vi "Main.vi"(7 "sweep rate, /min":dbl=0.2, 8 "sweep to:":dbl=-0.5, 9 "sweep":T3(radio)=enum."time_sweep") -> ()   [LabVIEW 2017] (continued)
                n2113 = property on="data_caption" class="Str"() -> ("Value"=w2662:string)  [unwired: 2 in, 2 out]
                n2114 = case shown="False" w2663 {
                  tunnel: w2662 -> [w2665 w2671]
                  tunnel: [w2665 w2670] -> w2661
                  tunnel: w2660 -> [w2664 w2668]
                  tunnel: [w2664 w2666] -> w2659
                  frame False {
                    # "not measure SR830 2 in phase signal (SR830_2_ip)"
                  }
                  frame True {
                    w2667 = "SR830_2_ip"
                    # "measure SR830 2 in phase signal (SR830_2_ip)"
                    n2115 = local read "SR830 2 addr"() -> (w2672:u8)
                    n2116 = Number To Decimal String(number=w2672) -> (decimal integer string=w2673:string)  [unwired: 1 in]
                    n2117 = GPIB Clear(3:w2673) -> ()  [unwired: 1 in, 2 out]
                    n2118 = Build Array (concatenate)(w2668, w2667) -> (w2666:string[])
                    n2119 = Concatenate Strings(w2671, w2667, "\t") -> (w2670:string)
                  }
                }
                n2120 = property on="Figure_axis" class="Arr (strict)"("Value"=w2659) -> ()  [unwired: 2 in, 2 out]
                n2121 = property on="data_caption" class="Str"("Value"=w2661) -> ()  [unwired: 2 in, 2 out]
              }
              frame #3 {
                # "SR830 2 out of phase (SR830_2_oop)"
                n2122 = local read "SR830 2 oop"() -> (w2678:bool)
                n2123 = property on="Figure_axis" class="Arr (strict)"() -> ("Value"=w2675:string[])  [unwired: 2 in, 2 out]
                n2124 = property on="data_caption" class="Str"() -> ("Value"=w2677:string)  [unwired: 2 in, 2 out]
                n2125 = case shown="False" w2678 {
                  tunnel: w2677 -> [w2680 w2686]
                  tunnel: [w2680 w2685] -> w2676
                  tunnel: w2675 -> [w2679 w2683]
                  tunnel: [w2679 w2681] -> w2674
                  frame False {
                    # "not measure SR830 2 out of phase signal (SR830_2_oop)"
                  }
                  frame True {
                    w2682 = "SR830_2_oop"
                    # "measure SR830 2 out of phase signal (SR830_2_oop)"
                    n2126 = local read "SR830 2 addr"() -> (w2687:u8)
                    n2127 = Number To Decimal String(number=w2687) -> (decimal integer string=w2688:string)  [unwired: 1 in]
                    n2128 = GPIB Clear(3:w2688) -> ()  [unwired: 1 in, 2 out]
                    n2129 = Build Array (concatenate)(w2683, w2682) -> (w2681:string[])
                    n2130 = Concatenate Strings(w2686, w2682, "\t") -> (w2685:string)
                  }
                }
                n2131 = property on="Figure_axis" class="Arr (strict)"("Value"=w2674) -> ()  [unwired: 2 in, 2 out]
                n2132 = property on="data_caption" class="Str"("Value"=w2676) -> ()  [unwired: 2 in, 2 out]
              }
              frame #4 {
                # "SR830 3 in phase (SR830_3_ip)"
                n2133 = local read "SR830 3 ip"() -> (w2693:bool)
                n2134 = property on="Figure_axis" class="Arr (strict)"() -> ("Value"=w2690:string[])  [unwired: 2 in, 2 out]
                n2135 = property on="data_caption" class="Str"() -> ("Value"=w2692:string)  [unwired: 2 in, 2 out]
                n2136 = case shown="False" w2693 {
                  tunnel: w2692 -> [w2695 w2701]
                  tunnel: [w2695 w2700] -> w2691
                  tunnel: w2690 -> [w2694 w2698]
                  tunnel: [w2694 w2696] -> w2689
                  frame False {
                    # "not measure SR830 3 in phase signal (SR830_3_ip)"
                  }
                  frame True {
                    w2697 = "SR830_3_ip"
                    # "measure SR830 3 in phase signal (SR830_3_ip)"
                    n2137 = local read "SR830 3 addr"() -> (w2702:u8)
                    n2138 = Number To Decimal String(number=w2702) -> (decimal integer string=w2703:string)  [unwired: 1 in]
                    n2139 = GPIB Clear(3:w2703) -> ()  [unwired: 1 in, 2 out]
                    n2140 = Build Array (concatenate)(w2698, w2697) -> (w2696:string[])
                    n2141 = Concatenate Strings(w2701, w2697, "\t") -> (w2700:string)
                  }
                }
                n2142 = property on="Figure_axis" class="Arr (strict)"("Value"=w2689) -> ()  [unwired: 2 in, 2 out]
                n2143 = property on="data_caption" class="Str"("Value"=w2691) -> ()  [unwired: 2 in, 2 out]
              }
              frame #5 {
                # "SR830 3 out of phase (SR830_3_oop)"
                n2144 = local read "SR830 3 oop"() -> (w2708:bool)
                n2145 = property on="Figure_axis" class="Arr (strict)"() -> ("Value"=w2705:string[])  [unwired: 2 in, 2 out]
                n2146 = property on="data_caption" class="Str"() -> ("Value"=w2707:string)  [unwired: 2 in, 2 out]
                n2147 = case shown="False" w2708 {
                  tunnel: w2707 -> [w2710 w2716]
                  tunnel: [w2710 w2715] -> w2706
                  tunnel: w2705 -> [w2709 w2713]
                  tunnel: [w2709 w2711] -> w2704
                  frame False {
                    # "not measure SR830 3 out of phase signal (SR830_3_oop)"
                  }
                  frame True {
                    w2712 = "SR830_3_oop"
                    # "measure SR830 3 out phase signal (SR830_3_oop)"
                    n2148 = local read "SR830 3 addr"() -> (w2717:u8)
                    n2149 = Number To Decimal String(number=w2717) -> (decimal integer string=w2718:string)  [unwired: 1 in]
                    n2150 = GPIB Clear(3:w2718) -> ()  [unwired: 1 in, 2 out]
                    n2151 = Build Array (concatenate)(w2713, w2712) -> (w2711:string[])
                    n2152 = Concatenate Strings(w2716, w2712, "\t") -> (w2715:string)
                  }
                }
                n2153 = property on="Figure_axis" class="Arr (strict)"("Value"=w2704) -> ()  [unwired: 2 in, 2 out]
                n2154 = property on="data_caption" class="Str"("Value"=w2706) -> ()  [unwired: 2 in, 2 out]
              }
              frame #6 {
                # "SR830 4 in phase (SR830_4_ip)"
                n2155 = local read "SR830 4 ip"() -> (w2723:bool)
                n2156 = property on="Figure_axis" class="Arr (strict)"() -> ("Value"=w2720:string[])  [unwired: 2 in, 2 out]
                n2157 = property on="data_caption" class="Str"() -> ("Value"=w2722:string)  [unwired: 2 in, 2 out]
                n2158 = case shown="False" w2723 {
                  tunnel: w2722 -> [w2725 w2731]
                  tunnel: [w2725 w2730] -> w2721
                  tunnel: w2720 -> [w2724 w2728]
                  tunnel: [w2724 w2726] -> w2719
                  frame False {
                    # "not measure SR830 4 in phase signal (SR830_4_ip)"
                  }
                  frame True {
                    w2727 = "SR830_4_ip"
                    # "measure SR830 4 in phase signal (SR830_4_ip)"
                    n2159 = local read "SR830 4 addr"() -> (w2732:u8)
                    n2160 = Number To Decimal String(number=w2732) -> (decimal integer string=w2733:string)  [unwired: 1 in]
                    n2161 = GPIB Clear(3:w2733) -> ()  [unwired: 1 in, 2 out]
                    n2162 = Build Array (concatenate)(w2728, w2727) -> (w2726:string[])
                    n2163 = Concatenate Strings(w2731, w2727, "\t") -> (w2730:string)
                  }
                }
                n2164 = property on="Figure_axis" class="Arr (strict)"("Value"=w2719) -> ()  [unwired: 2 in, 2 out]
                n2165 = property on="data_caption" class="Str"("Value"=w2721) -> ()  [unwired: 2 in, 2 out]
              }
              frame #7 {
                # "SR830 4 out of phase (SR830_4_oop)"
                n2166 = local read "SR830 4 oop"() -> (w2738:bool)
                n2167 = property on="Figure_axis" class="Arr (strict)"() -> ("Value"=w2735:string[])  [unwired: 2 in, 2 out]
                n2168 = property on="data_caption" class="Str"() -> ("Value"=w2737:string)  [unwired: 2 in, 2 out]
                n2169 = case shown="False" w2738 {
                  tunnel: w2737 -> [w2740 w2746]
                  tunnel: [w2740 w2745] -> w2736
                  tunnel: w2735 -> [w2739 w2743]
                  tunnel: [w2739 w2741] -> w2734
                  frame False {
                    # "not measure SR830 4 out of phase signal (SR830_4_oop)"
                  }
                  frame True {
                    w2742 = "SR830_4_oop"
                    # "measure SR830 4 out of phase signal (SR830_4_oop)"
                    n2170 = local read "SR830 4 addr"() -> (w2747:u8)
                    n2171 = Number To Decimal String(number=w2747) -> (decimal integer string=w2748:string)  [unwired: 1 in]
                    n2172 = GPIB Clear(3:w2748) -> ()  [unwired: 1 in, 2 out]
                    n2173 = Build Array (concatenate)(w2743, w2742) -> (w2741:string[])
                    n2174 = Concatenate Strings(w2746, w2742, "\t") -> (w2745:string)
                  }
                }
                n2175 = property on="Figure_axis" class="Arr (strict)"("Value"=w2734) -> ()  [unwired: 2 in, 2 out]
                n2176 = property on="data_caption" class="Str"("Value"=w2736) -> ()  [unwired: 2 in, 2 out]
              }
              frame #8 {
                # "2400 1 voltage measure (2400_1_v)"
                n2177 = local read "2400 1 meas v"() -> (w2753:bool)
                n2178 = property on="Figure_axis" class="Arr (strict)"() -> ("Value"=w2750:string[])  [unwired: 2 in, 2 out]
                n2179 = property on="data_caption" class="Str"() -> ("Value"=w2752:string)  [unwired: 2 in, 2 out]
                n2180 = case shown="False" w2753 {
                  tunnel: w2752 -> [w2755 w2761]
                  tunnel: [w2755 w2760] -> w2751
                  tunnel: w2750 -> [w2754 w2758]
                  tunnel: [w2754 w2756] -> w2749
                  frame False {
                    # "not measure 2400 1 voltage (2400_1_v)"
                  }
                  frame True {
                    w2757 = "2400_1_v"
                    # "measure 2400 1 voltage (2400_1_v)"
                    n2181 = local read "2400 1 addr"() -> (w2762:u8)
                    n2182 = Number To Decimal String(number=w2762) -> (decimal integer string=w2763:string)  [unwired: 1 in]
                    n2183 = GPIB Clear(3:w2763) -> ()  [unwired: 1 in, 2 out]
                    n2184 = Build Array (concatenate)(w2758, w2757) -> (w2756:string[])
                    n2185 = Concatenate Strings(w2761, w2757, "\t") -> (w2760:string)
                  }
                }
                n2186 = property on="Figure_axis" class="Arr (strict)"("Value"=w2749) -> ()  [unwired: 2 in, 2 out]
                n2187 = property on="data_caption" class="Str"("Value"=w2751) -> ()  [unwired: 2 in, 2 out]
              }
              frame #9 {
                # "2400 1 current measure (2400_1_i)"
                n2188 = local read "2400 1 meas i"() -> (w2768:bool)
                n2189 = property on="Figure_axis" class="Arr (strict)"() -> ("Value"=w2765:string[])  [unwired: 2 in, 2 out]
                n2190 = property on="data_caption" class="Str"() -> ("Value"=w2767:string)  [unwired: 2 in, 2 out]
                n2191 = case shown="False" w2768 {
                  tunnel: w2767 -> [w2770 w2776]
                  tunnel: [w2770 w2775] -> w2766
                  tunnel: w2765 -> [w2769 w2773]
                  tunnel: [w2769 w2771] -> w2764
                  frame False {
                    # "not measure 2400 1 current (2400_1_i)"
                  }
                  frame True {
                    w2772 = "2400_1_i"
                    # "measure 2400 1 current (2400_1_i)"
                    n2192 = local read "2400 1 addr"() -> (w2777:u8)
                    n2193 = Number To Decimal String(number=w2777) -> (decimal integer string=w2778:string)  [unwired: 1 in]
                    n2194 = GPIB Clear(3:w2778) -> ()  [unwired: 1 in, 2 out]
                    n2195 = Build Array (concatenate)(w2773, w2772) -> (w2771:string[])
                    n2196 = Concatenate Strings(w2776, w2772, "\t") -> (w2775:string)
                  }
                }
                n2197 = property on="Figure_axis" class="Arr (strict)"("Value"=w2764) -> ()  [unwired: 2 in, 2 out]
                n2198 = property on="data_caption" class="Str"("Value"=w2766) -> ()  [unwired: 2 in, 2 out]
              }
              frame #10 {
                # "2400 2 voltage measure (2400_2_v)"
                n2199 = local read "2400 2 meas v"() -> (w2783:bool)
                n2200 = property on="Figure_axis" class="Arr (strict)"() -> ("Value"=w2780:string[])  [unwired: 2 in, 2 out]
                n2201 = property on="data_caption" class="Str"() -> ("Value"=w2782:string)  [unwired: 2 in, 2 out]
                n2202 = case shown="False" w2783 {
                  tunnel: w2782 -> [w2785 w2791]
                  tunnel: [w2785 w2790] -> w2781
                  tunnel: w2780 -> [w2784 w2788]
                  tunnel: [w2784 w2786] -> w2779
                  frame False {
                    # "not measure 2400 2 voltage (2400_2_v)"
                  }
                  frame True {
                    w2787 = "2400_2_v"
                    # "measure 2400 2 voltage (2400_2_v)"
                    n2203 = local read "2400 2 addr"() -> (w2792:u8)
                    n2204 = Number To Decimal String(number=w2792) -> (decimal integer string=w2793:string)  [unwired: 1 in]
                    n2205 = GPIB Clear(3:w2793) -> ()  [unwired: 1 in, 2 out]
                    n2206 = Build Array (concatenate)(w2788, w2787) -> (w2786:string[])
                    n2207 = Concatenate Strings(w2791, w2787, "\t") -> (w2790:string)
                  }
                }
                n2208 = property on="Figure_axis" class="Arr (strict)"("Value"=w2779) -> ()  [unwired: 2 in, 2 out]
                n2209 = property on="data_caption" class="Str"("Value"=w2781) -> ()  [unwired: 2 in, 2 out]
              }
              frame #11 {
                # "2400 2 current measure (2400_2_i)"
                n2210 = local read "2400 2 meas i"() -> (w2798:bool)
                n2211 = property on="Figure_axis" class="Arr (strict)"() -> ("Value"=w2795:string[])  [unwired: 2 in, 2 out]
                n2212 = property on="data_caption" class="Str"() -> ("Value"=w2797:string)  [unwired: 2 in, 2 out]
                n2213 = case shown="False" w2798 {
                  tunnel: w2797 -> [w2800 w2806]
                  tunnel: [w2800 w2805] -> w2796
                  tunnel: w2795 -> [w2799 w2803]
                  tunnel: [w2799 w2801] -> w2794
                  frame False {
                    # "not measure 2400 2 current (2400_2_i)"
                  }
                  frame True {
                    w2802 = "2400_2_i"
                    # "measure 2400 2 current (2400_2_i)"
                    n2214 = local read "2400 2 addr"() -> (w2807:u8)
                    n2215 = Number To Decimal String(number=w2807) -> (decimal integer string=w2808:string)  [unwired: 1 in]
                    n2216 = GPIB Clear(3:w2808) -> ()  [unwired: 1 in, 2 out]
                    n2217 = Build Array (concatenate)(w2803, w2802) -> (w2801:string[])
                    n2218 = Concatenate Strings(w2806, w2802, "\t") -> (w2805:string)
                  }
                }
                n2219 = property on="Figure_axis" class="Arr (strict)"("Value"=w2794) -> ()  [unwired: 2 in, 2 out]
                n2220 = property on="data_caption" class="Str"("Value"=w2796) -> ()  [unwired: 2 in, 2 out]
              }
              frame #12 {
                # "2400 3 voltage measure (2400_3_v)"
                n2221 = local read "2400 3 meas v"() -> (w2813:bool)
                n2222 = property on="Figure_axis" class="Arr (strict)"() -> ("Value"=w2810:string[])  [unwired: 2 in, 2 out]
                n2223 = property on="data_caption" class="Str"() -> ("Value"=w2812:string)  [unwired: 2 in, 2 out]
                n2224 = case shown="False" w2813 {
                  tunnel: w2812 -> [w2815 w2821]
                  tunnel: [w2815 w2820] -> w2811
                  tunnel: w2810 -> [w2814 w2818]
                  tunnel: [w2814 w2816] -> w2809
                  frame False {
                    # "not measure 2400 3 voltage (2400_3_v)"
                  }
                  frame True {
                    w2817 = "2400_3_v"
                    # "measure 2400 3 voltage (2400_3_v)"
                    n2225 = local read "2400 3 addr"() -> (w2822:u8)
                    n2226 = Number To Decimal String(number=w2822) -> (decimal integer string=w2823:string)  [unwired: 1 in]
                    n2227 = GPIB Clear(3:w2823) -> ()  [unwired: 1 in, 2 out]
                    n2228 = Build Array (concatenate)(w2818, w2817) -> (w2816:string[])
                    n2229 = Concatenate Strings(w2821, w2817, "\t") -> (w2820:string)
                  }
                }
                n2230 = property on="Figure_axis" class="Arr (strict)"("Value"=w2809) -> ()  [unwired: 2 in, 2 out]
                n2231 = property on="data_caption" class="Str"("Value"=w2811) -> ()  [unwired: 2 in, 2 out]
              }
              frame #13 {
                # "2400 3 current measure (2400_3_i)"
                n2232 = local read "2400 3 meas i"() -> (w2828:bool)
                n2233 = property on="Figure_axis" class="Arr (strict)"() -> ("Value"=w2825:string[])  [unwired: 2 in, 2 out]
                n2234 = property on="data_caption" class="Str"() -> ("Value"=w2827:string)  [unwired: 2 in, 2 out]
                n2235 = case shown="True" w2828 {
                  tunnel: w2827 -> [w2830 w2836]
                  tunnel: [w2830 w2835] -> w2826
                  tunnel: w2825 -> [w2829 w2833]
                  tunnel: [w2829 w2831] -> w2824
                  frame False {
                    # "not measure 2400 3 current (2400_3_i)"
                  }
                  frame True {
                    w2832 = "2400_3_i"
                    # "measure 2400 3 current (2400_3_i)"
                    n2236 = local read "2400 3 addr"() -> (w2837:u8)
                    n2237 = Number To Decimal String(number=w2837) -> (decimal integer string=w2838:string)  [unwired: 1 in]
                    n2238 = GPIB Clear(3:w2838) -> ()  [unwired: 1 in, 2 out]
                    n2239 = Build Array (concatenate)(w2833, w2832) -> (w2831:string[])
                    n2240 = Concatenate Strings(w2836, w2832, "\t") -> (w2835:string)
                  }
                }
                n2241 = property on="Figure_axis" class="Arr (strict)"("Value"=w2824) -> ()  [unwired: 2 in, 2 out]
                n2242 = property on="data_caption" class="Str"("Value"=w2826) -> ()  [unwired: 2 in, 2 out]
              }
              frame #14 {
                # "2182A 1 channel 1 measure (2182A_1_ch1)"
                n2243 = local read "2182A 1 ch1"() -> (w2843:bool)
                n2244 = property on="Figure_axis" class="Arr (strict)"() -> ("Value"=w2840:string[])  [unwired: 2 in, 2 out]
                n2245 = property on="data_caption" class="Str"() -> ("Value"=w2842:string)  [unwired: 2 in, 2 out]
                n2246 = case shown="False" w2843 {
                  tunnel: w2842 -> [w2845 w2851]
                  tunnel: [w2845 w2850] -> w2841
                  tunnel: w2840 -> [w2844 w2848]
                  tunnel: [w2844 w2846] -> w2839
                  frame False {
                    # "not measure 2182A 1 channel 1 (2182A_1_ch1)"
                  }
                  frame True {
                    w2847 = "2182A_1_ch1"
                    # "measure 2182A 1 channel 1 (2182A_1_ch1)"
                    n2247 = local read "2182A 1 addr"() -> (w2852:u8)
                    n2248 = Number To Decimal String(number=w2852) -> (decimal integer string=w2853:string)  [unwired: 1 in]
                    n2249 = GPIB Clear(3:w2853) -> ()  [unwired: 1 in, 2 out]
                    n2250 = Build Array (concatenate)(w2848, w2847) -> (w2846:string[])
                    n2251 = Concatenate Strings(w2851, w2847, "\t") -> (w2850:string)
                  }
                }
                n2252 = property on="Figure_axis" class="Arr (strict)"("Value"=w2839) -> ()  [unwired: 2 in, 2 out]
                n2253 = property on="data_caption" class="Str"("Value"=w2841) -> ()  [unwired: 2 in, 2 out]
              }
              frame #15 {
                # "2182A 1 channel 2 measure (2182A_1_ch2)"
                n2254 = local read "2182A 1 ch2"() -> (w2858:bool)
                n2255 = property on="Figure_axis" class="Arr (strict)"() -> ("Value"=w2855:string[])  [unwired: 2 in, 2 out]
                n2256 = property on="data_caption" class="Str"() -> ("Value"=w2857:string)  [unwired: 2 in, 2 out]
                n2257 = case shown="True" w2858 {
                  tunnel: w2857 -> [w2860 w2866]
                  tunnel: [w2860 w2865] -> w2856
                  tunnel: w2855 -> [w2859 w2863]
                  tunnel: [w2859 w2861] -> w2854
                  frame False {
                    # "not measure 2182A 1 channel 2 (2182A_1_ch2)"
                  }
                  frame True {
                    w2862 = "2182A_1_ch2"
                    # "measure 2182A 1 channel 2 (2182A_1_ch2)"
                    n2258 = local read "2182A 1 addr"() -> (w2867:u8)
                    n2259 = Number To Decimal String(number=w2867) -> (decimal integer string=w2868:string)  [unwired: 1 in]
                    n2260 = GPIB Clear(3:w2868) -> ()  [unwired: 1 in, 2 out]
                    n2261 = Build Array (concatenate)(w2863, w2862) -> (w2861:string[])
                    n2262 = Concatenate Strings(w2866, w2862, "\t") -> (w2865:string)
                  }
                }
                n2263 = property on="Figure_axis" class="Arr (strict)"("Value"=w2854) -> ()  [unwired: 2 in, 2 out]
                n2264 = property on="data_caption" class="Str"("Value"=w2856) -> ()  [unwired: 2 in, 2 out]
              }
              frame #16 {
                # "2182A 2 channel 1 measure (2182A_2_ch1)"
                n2265 = local read "2182A 2 ch1"() -> (w2873:bool)
                n2266 = property on="Figure_axis" class="Arr (strict)"() -> ("Value"=w2870:string[])  [unwired: 2 in, 2 out]
                n2267 = property on="data_caption" class="Str"() -> ("Value"=w2872:string)  [unwired: 2 in, 2 out]
                n2268 = case shown="True" w2873 {
                  tunnel: w2872 -> [w2875 w2881]
                  tunnel: [w2875 w2880] -> w2871
                  tunnel: w2870 -> [w2874 w2878]
                  tunnel: [w2874 w2876] -> w2869
                  frame False {
                    # "not measure 2182A 2 channel 1 (2182A_2_ch1)"
                  }
                  frame True {
                    w2877 = "2182A_2_ch1"
                    # "measure 2182A 2 channel 1 (2182A_2_ch1)"
                    n2269 = local read "2182A 2 addr"() -> (w2882:u8)
                    n2270 = Number To Decimal String(number=w2882) -> (decimal integer string=w2883:string)  [unwired: 1 in]
                    n2271 = GPIB Clear(3:w2883) -> ()  [unwired: 1 in, 2 out]
                    n2272 = Build Array (concatenate)(w2878, w2877) -> (w2876:string[])
                    n2273 = Concatenate Strings(w2881, w2877, "\t") -> (w2880:string)
                  }
                }
                n2274 = property on="Figure_axis" class="Arr (strict)"("Value"=w2869) -> ()  [unwired: 2 in, 2 out]
                n2275 = property on="data_caption" class="Str"("Value"=w2871) -> ()  [unwired: 2 in, 2 out]
              }
              frame #17 {
                # "2182A 2 channel 2 measure (2182A_2_ch2)"
                n2276 = local read "2182A 2 ch2"() -> (w2888:bool)
                n2277 = property on="Figure_axis" class="Arr (strict)"() -> ("Value"=w2885:string[])  [unwired: 2 in, 2 out]
                n2278 = property on="data_caption" class="Str"() -> ("Value"=w2887:string)  [unwired: 2 in, 2 out]
                n2279 = case shown="True" w2888 {
                  tunnel: w2887 -> [w2890 w2896]
                  tunnel: [w2890 w2895] -> w2886
                  tunnel: w2885 -> [w2889 w2893]
                  tunnel: [w2889 w2891] -> w2884
                  frame False {
                    # "not measure 2182A 2 channel 2 (2182A_2_ch2)"
                  }
                  frame True {
                    w2892 = "2182A_2_ch2"
                    # "measure 2182A 2 channel 2 (2182A_2_ch2)"
                    n2280 = local read "2182A 2 addr"() -> (w2897:u8)
                    n2281 = Number To Decimal String(number=w2897) -> (decimal integer string=w2898:string)  [unwired: 1 in]
                    n2282 = GPIB Clear(3:w2898) -> ()  [unwired: 1 in, 2 out]
                    n2283 = Build Array (concatenate)(w2893, w2892) -> (w2891:string[])
                    n2284 = Concatenate Strings(w2896, w2892, "\t") -> (w2895:string)
                  }
                }
                n2285 = property on="Figure_axis" class="Arr (strict)"("Value"=w2884) -> ()  [unwired: 2 in, 2 out]
                n2286 = property on="data_caption" class="Str"("Value"=w2886) -> ()  [unwired: 2 in, 2 out]
              }
              frame #18 {
                # "2182A 3 channel 1 measure (2182A_3_ch1)"
                n2287 = local read "2182A 3 ch1"() -> (w2903:bool)
                n2288 = property on="Figure_axis" class="Arr (strict)"() -> ("Value"=w2900:string[])  [unwired: 2 in, 2 out]
                n2289 = property on="data_caption" class="Str"() -> ("Value"=w2902:string)  [unwired: 2 in, 2 out]
                n2290 = case shown="True" w2903 {
                  tunnel: w2902 -> [w2905 w2911]
                  tunnel: [w2905 w2910] -> w2901
                  tunnel: w2900 -> [w2904 w2908]
                  tunnel: [w2904 w2906] -> w2899
                  frame False {
                    # "not measure 2182A 3 channel 1 (2182A_3_ch1)"
                  }
                  frame True {
                    w2907 = "2182A_3_ch1"
                    # "measure 2182A 3 channel 1 (2182A_3_ch1)"
                    n2291 = local read "2182A 3 addr"() -> (w2912:u8)
                    n2292 = Number To Decimal String(number=w2912) -> (decimal integer string=w2913:string)  [unwired: 1 in]
                    n2293 = GPIB Clear(3:w2913) -> ()  [unwired: 1 in, 2 out]
                    n2294 = Build Array (concatenate)(w2908, w2907) -> (w2906:string[])
                    n2295 = Concatenate Strings(w2911, w2907, "\t") -> (w2910:string)
                  }
                }
                n2296 = property on="Figure_axis" class="Arr (strict)"("Value"=w2899) -> ()  [unwired: 2 in, 2 out]
                n2297 = property on="data_caption" class="Str"("Value"=w2901) -> ()  [unwired: 2 in, 2 out]
              }
              frame #19 {
                # "2182A 3 channel 2 measure (2182A_3_ch2)"
                n2298 = local read "2182A 3 ch2"() -> (w2918:bool)
                n2299 = property on="Figure_axis" class="Arr (strict)"() -> ("Value"=w2915:string[])  [unwired: 2 in, 2 out]
                n2300 = property on="data_caption" class="Str"() -> ("Value"=w2917:string)  [unwired: 2 in, 2 out]
                n2301 = case shown="False" w2918 {
                  tunnel: w2917 -> [w2920 w2926]
                  tunnel: [w2920 w2925] -> w2916
                  tunnel: w2915 -> [w2919 w2923]
                  tunnel: [w2919 w2921] -> w2914
                  frame False {
                    # "not measure 2182A 3 channel 2 (2182A_3_ch2)"
                  }
                  frame True {
                    w2922 = "2182A_3_ch2"
                    # "measure 2182A 3 channel 2 (2182A_3_ch2)"
                    n2302 = local read "2182A 3 addr"() -> (w2927:u8)
                    n2303 = Number To Decimal String(number=w2927) -> (decimal integer string=w2928:string)  [unwired: 1 in]
                    n2304 = GPIB Clear(3:w2928) -> ()  [unwired: 1 in, 2 out]
                    n2305 = Build Array (concatenate)(w2923, w2922) -> (w2921:string[])
                    n2306 = Concatenate Strings(w2926, w2922, "\t") -> (w2925:string)
                  }
                }
                n2307 = property on="Figure_axis" class="Arr (strict)"("Value"=w2914) -> ()  [unwired: 2 in, 2 out]
                n2308 = property on="data_caption" class="Str"("Value"=w2916) -> ()  [unwired: 2 in, 2 out]
              }
              frame #20 {
                # "2182A 4 channel 1 measure (2182A_4_ch1)"
                n2309 = local read "2182A 4 ch1"() -> (w2933:bool)
                n2310 = property on="Figure_axis" class="Arr (strict)"() -> ("Value"=w2930:string[])  [unwired: 2 in, 2 out]
                n2311 = property on="data_caption" class="Str"() -> ("Value"=w2932:string)  [unwired: 2 in, 2 out]
                n2312 = case shown="True" w2933 {
                  tunnel: w2932 -> [w2935 w2941]
                  tunnel: [w2935 w2940] -> w2931
                  tunnel: w2930 -> [w2934 w2938]
                  tunnel: [w2934 w2936] -> w2929
                  frame False {
                    # "not measure 2182A 4 channel 1 (2182A_4_ch1)"
                  }
                  frame True {
                    w2937 = "2182A_4_ch1"
                    # "measure 2182A 4 channel 1 (2182A_4_ch1)"
                    n2313 = local read "2182A 4 addr"() -> (w2942:u8)
                    n2314 = Number To Decimal String(number=w2942) -> (decimal integer string=w2943:string)  [unwired: 1 in]
                    n2315 = GPIB Clear(3:w2943) -> ()  [unwired: 1 in, 2 out]
                    n2316 = Build Array (concatenate)(w2938, w2937) -> (w2936:string[])
                    n2317 = Concatenate Strings(w2941, w2937, "\t") -> (w2940:string)
                  }
                }
                n2318 = property on="Figure_axis" class="Arr (strict)"("Value"=w2929) -> ()  [unwired: 2 in, 2 out]
                n2319 = property on="data_caption" class="Str"("Value"=w2931) -> ()  [unwired: 2 in, 2 out]
              }
              frame #21 {
                # "2182A 4 channel 2 measure (2182A_4_ch2)"
                n2320 = local read "2182A 4 ch2"() -> (w2948:bool)
                n2321 = property on="Figure_axis" class="Arr (strict)"() -> ("Value"=w2945:string[])  [unwired: 2 in, 2 out]
                n2322 = property on="data_caption" class="Str"() -> ("Value"=w2947:string)  [unwired: 2 in, 2 out]
                n2323 = case shown="True" w2948 {
                  tunnel: w2947 -> [w2950 w2956]
                  tunnel: [w2950 w2955] -> w2946
                  tunnel: w2945 -> [w2949 w2953]
                  tunnel: [w2949 w2951] -> w2944
                  frame False {
                    # "not measure 2182A 4 channel 2 (2182A_4_ch2)"
                  }
                  frame True {
                    w2952 = "2182A_4_ch2"
                    # "measure 2182A 4 channel 2 (2182A_4_ch2)"
                    n2324 = local read "2182A 4 addr"() -> (w2957:u8)
                    n2325 = Number To Decimal String(number=w2957) -> (decimal integer string=w2958:string)  [unwired: 1 in]
                    n2326 = GPIB Clear(3:w2958) -> ()  [unwired: 1 in, 2 out]
                    n2327 = Build Array (concatenate)(w2953, w2952) -> (w2951:string[])
                    n2328 = Concatenate Strings(w2956, w2952, "\t") -> (w2955:string)
                  }
                }
                n2329 = property on="Figure_axis" class="Arr (strict)"("Value"=w2944) -> ()  [unwired: 2 in, 2 out]
                n2330 = property on="data_caption" class="Str"("Value"=w2946) -> ()  [unwired: 2 in, 2 out]
              }
              frame #22 {
                # "2636A smua measure voltage (2636A_smua_v)"
                n2331 = local read "2636A smua meas v"() -> (w2963:bool)
                n2332 = property on="Figure_axis" class="Arr (strict)"() -> ("Value"=w2960:string[])  [unwired: 2 in, 2 out]
                n2333 = property on="data_caption" class="Str"() -> ("Value"=w2962:string)  [unwired: 2 in, 2 out]
                n2334 = case shown="True" w2963 {
                  tunnel: w2962 -> [w2965 w2976]
                  tunnel: [w2965 w2975] -> w2961
                  tunnel: w2960 -> [w2964 w2973]
                  tunnel: [w2964 w2971] -> w2959
                  frame False {
                    # "not measure voltage on 2636A smua (2636A_smua_v)"
                  }
                  frame True {
                    w2972 = "2636A_smua_v"
                    # "measure voltage on 2636A smua (2636A_smua_v)"
                    n2335 = local read "2336A addr"() -> (w2967:refnum<visa-resource-name>)
                    n2336 = VISA Open(VISA resource name=w2967) -> (VISA resource name=w2966:refnum<visa-resource-name>, error out=w2968:errorcluster)  [unwired: 4 in]
                    n2337 = VISA Clear(VISA resource name=w2966, error in (no error)=w2968) -> (VISA resource name out=w2970:refnum<visa-resource-name>)  [unwired: 1 out]
                    n2338 = property class="Instr"(reference=w2970, "General Settings:Timeout Value"=u32 10000) -> ()  [unwired: 1 in, 2 out]
                    n2339 = Build Array (concatenate)(w2973, w2972) -> (w2971:string[])
                    n2340 = Concatenate Strings(w2976, w2972, "\t") -> (w2975:string)
                  }
                }
                n2341 = property on="Figure_axis" class="Arr (strict)"("Value"=w2959) -> ()  [unwired: 2 in, 2 out]
                n2342 = property on="data_caption" class="Str"("Value"=w2961) -> ()  [unwired: 2 in, 2 out]
              }
              frame #23 {
                # "2636A smua measure current (2636A_smua_i)"
                n2343 = local read "2636A smua meas i"() -> (w2981:bool)
                n2344 = property on="Figure_axis" class="Arr (strict)"() -> ("Value"=w2978:string[])  [unwired: 2 in, 2 out]
                n2345 = property on="data_caption" class="Str"() -> ("Value"=w2980:string)  [unwired: 2 in, 2 out]
                n2346 = case shown="True" w2981 {
                  tunnel: w2980 -> [w2983 w2994]
                  tunnel: [w2983 w2993] -> w2979
                  tunnel: w2978 -> [w2982 w2991]
                  tunnel: [w2982 w2989] -> w2977
                  frame False {
                    # "not measure current on 2636A smua (2636A_smua_i)"
                  }
                  frame True {
                    w2990 = "2636A_smua_i"
                    # "measure current on 2636A smua (2636A_smua_i)"
                    n2347 = local read "2336A addr"() -> (w2986:refnum<visa-resource-name>)
                    n2348 = VISA Open(VISA resource name=w2986) -> (VISA resource name=w2985:refnum<visa-resource-name>, error out=w2984:errorcluster)  [unwired: 4 in]
                    n2349 = VISA Clear(VISA resource name=w2985, error in (no error)=w2984) -> (VISA resource name out=w2987:refnum<visa-resource-name>)  [unwired: 1 out]
                    n2350 = Build Array (concatenate)(w2991, w2990) -> (w2989:string[])
                    n2351 = property class="Instr"(reference=w2987, "General Settings:Timeout Value"=u32 10000) -> ()  [unwired: 1 in, 2 out]
                    n2352 = Concatenate Strings(w2994, w2990, "\t") -> (w2993:string)
                  }
                }
                n2353 = property on="Figure_axis" class="Arr (strict)"("Value"=w2977) -> ()  [unwired: 2 in, 2 out]
                n2354 = property on="data_caption" class="Str"("Value"=w2979) -> ()  [unwired: 2 in, 2 out]
              }
              frame #24 {
                # "2636A smub measure voltage (2636A_smub_v)"
                n2355 = local read "2636A smub meas v"() -> (w2999:bool)
                n2356 = property on="Figure_axis" class="Arr (strict)"() -> ("Value"=w2996:string[])  [unwired: 2 in, 2 out]
                n2357 = property on="data_caption" class="Str"() -> ("Value"=w2998:string)  [unwired: 2 in, 2 out]
                n2358 = case shown="True" w2999 {
                  tunnel: w2998 -> [w3001 w3012]
                  tunnel: [w3001 w3011] -> w2997
                  tunnel: w2996 -> [w3000 w3009]
                  tunnel: [w3000 w3007] -> w2995
                  frame False {
                    # "not measure voltage on 2636A smub (2636A_smub_v)"
                  }
                  frame True {
                    w3008 = "2636A_smub_v"
                    # "measure voltage on 2636A smub (2636A_smub_v)"
                    n2359 = local read "2336A addr"() -> (w3003:refnum<visa-resource-name>)
                    n2360 = VISA Open(VISA resource name=w3003) -> (VISA resource name=w3002:refnum<visa-resource-name>, error out=w3004:errorcluster)  [unwired: 4 in]
                    n2361 = VISA Clear(VISA resource name=w3002, error in (no error)=w3004) -> (VISA resource name out=w3005:refnum<visa-resource-name>)  [unwired: 1 out]
                    n2362 = Build Array (concatenate)(w3009, w3008) -> (w3007:string[])
                    n2363 = property class="Instr"(reference=w3005, "General Settings:Timeout Value"=u32 10000) -> ()  [unwired: 1 in, 2 out]
                    n2364 = Concatenate Strings(w3012, w3008, "\t") -> (w3011:string)
                  }
                }
                n2365 = property on="Figure_axis" class="Arr (strict)"("Value"=w2995) -> ()  [unwired: 2 in, 2 out]
                n2366 = property on="data_caption" class="Str"("Value"=w2997) -> ()  [unwired: 2 in, 2 out]
              }
              frame #25 {
                # "2636A smub measure current (2636A_smub_i)"
                n2367 = local read "2636A smub meas i"() -> (w3017:bool)
                n2368 = property on="Figure_axis" class="Arr (strict)"() -> ("Value"=w3014:string[])  [unwired: 2 in, 2 out]
                n2369 = property on="data_caption" class="Str"() -> ("Value"=w3016:string)  [unwired: 2 in, 2 out]
                n2370 = case shown="True" w3017 {
                  tunnel: w3016 -> [w3019 w3030]
                  tunnel: [w3019 w3029] -> w3015
                  tunnel: w3014 -> [w3018 w3027]
                  tunnel: [w3018 w3025] -> w3013
                  frame False {
                    # "not measure current on 2636A smub (2636A_smub_i)"
                  }
                  frame True {
                    w3026 = "2636A_smub_i"
                    # "measure current on 2636A smub (2636A_smub_i)"
                    n2371 = local read "2336A addr"() -> (w3020:refnum<visa-resource-name>)
                    n2372 = VISA Open(VISA resource name=w3020) -> (VISA resource name=w3021:refnum<visa-resource-name>, error out=w3022:errorcluster)  [unwired: 4 in]
                    n2373 = VISA Clear(VISA resource name=w3021, error in (no error)=w3022) -> (VISA resource name out=w3023:refnum<visa-resource-name>)  [unwired: 1 out]
                    n2374 = Build Array (concatenate)(w3027, w3026) -> (w3025:string[])
                    n2375 = property class="Instr"(reference=w3023, "General Settings:Timeout Value"=u32 10000) -> ()  [unwired: 1 in, 2 out]
                    n2376 = Concatenate Strings(w3030, w3026, "\t") -> (w3029:string)
                  }
                }
                n2377 = property on="Figure_axis" class="Arr (strict)"("Value"=w3013) -> ()  [unwired: 2 in, 2 out]
                n2378 = property on="data_caption" class="Str"("Value"=w3015) -> ()  [unwired: 2 in, 2 out]
              }
              frame #26 {
                # "measure time"
                n2379 = local read "measure time"() -> (w3035:bool)
                n2380 = property on="Figure_axis" class="Arr (strict)"() -> ("Value"=w3032:string[])  [unwired: 2 in, 2 out]
                n2381 = property on="data_caption" class="Str"() -> ("Value"=w3034:string)  [unwired: 2 in, 2 out]
                n2382 = case shown="True" w3035 {
                  tunnel: w3034 -> [w3037 w3043]
                  tunnel: [w3037 w3042] -> w3033
                  tunnel: w3032 -> [w3036 w3040]
                  tunnel: [w3036 w3038] -> w3031
                  frame False {
                    # "not measuring time"
                  }
                  frame True {
                    w3039 = "time"
                    # "measuring time"
                    n2383 = Build Array (concatenate)(w3040, w3039) -> (w3038:string[])
                    n2384 = Concatenate Strings(w3043, w3039, "\t") -> (w3042:string)
                  }
                }
                n2385 = property on="Figure_axis" class="Arr (strict)"("Value"=w3031) -> ()  [unwired: 2 in, 2 out]
                n2386 = property on="data_caption" class="Str"("Value"=w3033) -> ()  [unwired: 2 in, 2 out]
              }
              frame #27 {
                # "Measure magnetic field on IPS120-0"
                n2387 = local read "iPS_MagnetField"() -> (w3048:bool)
                n2388 = property on="Figure_axis" class="Arr (strict)"() -> ("Value"=w3045:string[])  [unwired: 2 in, 2 out]
                n2389 = property on="data_caption" class="Str"() -> ("Value"=w3047:string)  [unwired: 2 in, 2 out]
                n2390 = case shown="True" w3048 {
                  tunnel: w3047 -> [w3050 w3056]
                  tunnel: [w3050 w3055] -> w3046
                  tunnel: w3045 -> [w3049 w3053]
                  tunnel: [w3049 w3051] -> w3044
                  frame False {
                    # "do not Measure magnetic field on IPS120-0"
                  }
                  frame True {
                    w3052 = "iPS_MagntField"
                    n2391 = Build Array (concatenate)(w3053, w3052) -> (w3051:string[])
                    n2392 = Concatenate Strings(w3056, w3052, "\t") -> (w3055:string)
                  }
                }
                n2393 = property on="Figure_axis" class="Arr (strict)"("Value"=w3044) -> ()  [unwired: 2 in, 2 out]
                n2394 = property on="data_caption" class="Str"("Value"=w3046) -> ()  [unwired: 2 in, 2 out]
              }
              frame #28 {
                # "iTC sample Temp"
                n2395 = property on="iTC_Sample_T" class="Bool (strict)"() -> ("Value"=w3057:bool)  [unwired: 2 in, 2 out]
                n2396 = property on="Figure_axis" class="Arr (strict)"() -> ("Value"=w3059:string[])  [unwired: 2 in, 2 out]
                n2397 = property on="data_caption" class="Str"() -> ("Value"=w3061:string)  [unwired: 2 in, 2 out]
                n2398 = case shown="True" w3057 {
                  tunnel: w3061 -> [w3063 w3069]
                  tunnel: [w3063 w3068] -> w3060
                  tunnel: w3059 -> [w3062 w3066]
                  tunnel: [w3062 w3064] -> w3058
                  frame False {
                    # "not measure 2461 voltage (2461_meas_v)"
                  }
                  frame True {
                    w3065 = "iTC_Sample_T"
                    n2399 = Build Array (concatenate)(w3066, w3065) -> (w3064:string[])
                    n2400 = Concatenate Strings(w3069, w3065, "\t") -> (w3068:string)
                  }
                }
                n2401 = property on="Figure_axis" class="Arr (strict)"("Value"=w3058) -> ()  [unwired: 2 in, 2 out]
                n2402 = property on="data_caption" class="Str"("Value"=w3060) -> ()  [unwired: 2 in, 2 out]
              }
              frame #29 {
                # "iTC sample Temp"
                n2403 = property on="CH_A" class="Bool (strict)"() -> ("Value"=w3070:bool)  [unwired: 2 in, 2 out]
                n2404 = property on="Figure_axis" class="Arr (strict)"() -> ("Value"=w3072:string[])  [unwired: 2 in, 2 out]
                n2405 = property on="data_caption" class="Str"() -> ("Value"=w3074:string)  [unwired: 2 in, 2 out]
                n2406 = case shown="True" w3070 {
                  tunnel: w3074 -> [w3076 w3082]
                  tunnel: [w3076 w3081] -> w3073
                  tunnel: w3072 -> [w3075 w3079]
                  tunnel: [w3075 w3077] -> w3071
                  frame False {
                    # "not measure 2461 voltage (2461_meas_v)"
                  }
                  frame True {
                    w3078 = "iTC_CHA_A"
                    n2407 = Build Array (concatenate)(w3079, w3078) -> (w3077:string[])
                    n2408 = Concatenate Strings(w3082, w3078, "\t") -> (w3081:string)
                  }
                }
                n2409 = property on="Figure_axis" class="Arr (strict)"("Value"=w3071) -> ()  [unwired: 2 in, 2 out]
                n2410 = property on="data_caption" class="Str"("Value"=w3073) -> ()  [unwired: 2 in, 2 out]
              }
              frame #30 {
                # "iTC sample Temp"
                n2411 = property on="CH_B" class="Bool (strict)"() -> ("Value"=w3083:bool)  [unwired: 2 in, 2 out]
                n2412 = property on="Figure_axis" class="Arr (strict)"() -> ("Value"=w3085:string[])  [unwired: 2 in, 2 out]
                n2413 = property on="data_caption" class="Str"() -> ("Value"=w3087:string)  [unwired: 2 in, 2 out]
                n2414 = case shown="True" w3083 {
                  tunnel: w3087 -> [w3089 w3095]
                  tunnel: [w3089 w3094] -> w3086
                  tunnel: w3085 -> [w3088 w3092]
                  tunnel: [w3088 w3090] -> w3084
                  frame False {
                    # "not measure 2461 voltage (2461_meas_v)"
                  }
                  frame True {
                    w3091 = "iTC_CH_B"
                    n2415 = Build Array (concatenate)(w3092, w3091) -> (w3090:string[])
                    n2416 = Concatenate Strings(w3095, w3091, "\t") -> (w3094:string)
                  }
                }
                n2417 = property on="Figure_axis" class="Arr (strict)"("Value"=w3084) -> ()  [unwired: 2 in, 2 out]
                n2418 = property on="data_caption" class="Str"("Value"=w3086) -> ()  [unwired: 2 in, 2 out]
              }
            }
          }
          frame #2 {
            # "1 = 2400 1\n2 = 2400 2\n3 = 2400 3\n4 = 2636a smua\n5 = 2636a smub\n6 = do not sweep, just time\n7 = Teslatron_iPS_Field\n8 = Teslatron_iTC_Sample T"
            n2419 = property on="sweep" class="RadioBtnsControl (strict)"() -> ("Value"=w3096:T3)  [unwired: 2 in, 2 out]
            n2420 = case "reads current value from instrument which will be sweeping" shown="\"2400_1\", Default" w3096 {
              tunnel: [w3098 w3108 w3117 w3126 w3130 0.0 ("Measuremet") w3136 w3137] -> w3097
              frame "2400_1", Default {
                # "reads the voltage on 2400 1"
                n2421 = local read "2400 1 addr"() -> (w3102:u8)
                n2422 = Number To Decimal String(number=w3102) -> (decimal integer string=w3103:string)  [unwired: 1 in]
                n2423 = GPIB Write(0:w3103, 1:":READ?") -> (6:w3099:errorcluster)  [unwired: 3 in, 1 out]
                n2424 = GPIB Read(0:w3103, 1:3200, 3:w3099) -> (5:w3105:string)  [unwired: 2 in, 2 out]
                n2425 = String Subset(string=w3105, length (rest)=13) -> (substring=w3106:string)  [unwired: 1 in]
                n2426 = Fract/Exp String To Number(string=w3106) -> (number=w3098:dbl)  [unwired: 3 in, 1 out]
              }
              frame "2400_2" {
                # "reads the current on 2400 2"
                n2427 = local read "2400 2 addr"() -> (w3112:u8)
                n2428 = Number To Decimal String(number=w3112) -> (decimal integer string=w3113:string)  [unwired: 1 in]
                n2429 = GPIB Write(0:w3113, 1:":READ?") -> (6:w3109:errorcluster)  [unwired: 3 in, 1 out]
                n2430 = GPIB Read(0:w3113, 1:3200, 3:w3109) -> (5:w3115:string)  [unwired: 2 in, 2 out]
                n2431 = String Subset(string=w3115, offset (0)=14, length (rest)=13) -> (substring=w3116:string)
                n2432 = Fract/Exp String To Number(string=w3116) -> (number=w3108:dbl)  [unwired: 3 in, 1 out]
              }
              frame "2400_3" {
                # "reads the voltage on 2400 3"
                n2433 = local read "2400 3 addr"() -> (w3121:u8)
                n2434 = Number To Decimal String(number=w3121) -> (decimal integer string=w3122:string)  [unwired: 1 in]
                n2435 = GPIB Write(0:w3122, 1:":READ?") -> (6:w3118:errorcluster)  [unwired: 3 in, 1 out]
                n2436 = GPIB Read(0:w3122, 1:3200, 3:w3118) -> (5:w3124:string)  [unwired: 2 in, 2 out]
                n2437 = String Subset(string=w3124, length (rest)=13) -> (substring=w3125:string)  [unwired: 1 in]
                n2438 = Fract/Exp String To Number(string=w3125) -> (number=w3117:dbl)  [unwired: 3 in, 1 out]
              }
              frame "2636a_smua" {
                # "reads the voltage on 2636a smua"
                n2439 = local read "2336A addr"() -> (w3129:refnum<visa-resource-name>)
                n2440 = call "SinglePointMeasurement.vi"("Measure"=Measure."Voltage", "Channel"=Channel."a", "VISA resource name 2"=w3129) -> ("Measuremet"=w3126:dbl)  [unwired: 3 in, 4 out]
              }
              frame "2636a_smub" {
                # "reads the voltage on 2636a smub"
                n2441 = local read "2336A addr"() -> (w3133:refnum<visa-resource-name>)
                n2442 = call "SinglePointMeasurement.vi"("Measure"=Measure."Voltage", "Channel"=Channel."b", "VISA resource name 2"=w3133) -> ("Measuremet"=w3130:dbl)  [unwired: 3 in, 4 out]
              }
              frame "time_sweep" {
              }
              frame "iPS" {
                # "Measure magnetic field on IPS120-0"
                n2443 = call "iPSread.vi"("iPSreadCtrl"=iPSreadCtrl."OutputField") -> ("number"=w3136:dbl)  [unwired: 7 in, 3 out]
              }
              frame "iTC" {
                n2444 = call "iTCread.vi"("iTCreadCtrl"=iTCreadCtrl."Sample Temp") -> ("number"=w3137:dbl)  [unwired: 6 in, 3 out]
              }
            }
          }
          frame #3 {
            # "add \"formula\" string to the axis rings"
            n2445 = property on="Figure_axis" class="Arr (strict)"() -> ("Value"=w3141:string[])  [unwired: 2 in, 2 out]
            n2446 = Build Array (concatenate)(w3141, "formula") -> (w3139:string[])
            n2447 = property on="Figure_axis" class="Arr (strict)"("Value"=w3139) -> ()  [unwired: 2 in, 2 out]
          }
          frame #4 {
            # "passes array to ring"
            n2448 = property on="Figure_axis" class="Arr (strict)"() -> ("Value"=w3143:string[])  [unwired: 2 in, 2 out]
            n2449 = property on="Xaxis" class="Ring (strict)"("Strings []"=w3143) -> ()  [unwired: 2 in, 2 out]
            n2450 = property on="Yright" class="Ring (strict)"("Strings []"=w3143) -> ()  [unwired: 2 in, 2 out]
            n2451 = property on="Yaxis" class="Ring (strict)"("Strings []"=w3143) -> ()  [unwired: 2 in, 2 out]
            n2452 = property on="Stop Ramp" class="Bool"("DisabledEnum"=T5."Enabled" ("Disabled")) -> ()  [unwired: 2 in, 2 out]
          }
        }
        n2453 = call "timeInSeconds.vi"() -> ("Numeric"=w2572:dbl)  [unwired: 2 in, 1 out]
        n2454 = while {
          shift-right: [w3173] -> w2571
          shift-left: w2569 -> [w3172]
          tunnel: w2572 -> [w3170]
          shift-right: [w3164] -> _
          shift-left: w2568 -> [w3165]
          stop <- w3168 stop-if-true
          # "initial value"
          # "this loop stops when target value is reached"
          n2455 = stacked-sequence {
            tunnel: [_ _ w3259 _ _] -> w3167
            tunnel: [_ _ w3258 _ _] -> w3174
            tunnel: w3172 -> [_ _ w3254 _ _]
            tunnel: [w3247 _ _ _ _] -> w3171
            tunnel: w3170 -> [_ _ _ w3274 _]
            tunnel: [_ _ w3254 _ _] -> w3169
            tunnel: [_ _ _ _ w3723] -> w3163
            frame #0 {
              # "time is measured at the beginning\nand at the end of the cycle to\ncalculate delay time required to\nkeep set sweep rate"
              n2456 = flat-sequence {
                tunnel: [w3249] -> w3247
                frame #0 {
                  n2457 = property on="time delay, ms" class="DigNum (strict)"() -> ("Value"=w3248:dbl)  [unwired: 2 in, 2 out]
                  n2458 = Wait (ms)(milliseconds to wait=w3248) -> ()  [unwired: 1 out]
                }
                frame #1 {
                  n2459 = Tick Count (ms)() -> (millisecond timer value=w3249:u32)
                }
              }
            }
            frame #1 {
              w3250 = dbl[] []  # Empty array for data
              # "clear data array before each measurement cycle"
              n2460 = property on="data" class="Arr (strict)"("Value"=w3250) -> ()  [unwired: 2 in, 2 out]
            }
            frame #2 {
              # "add next sweep value to the data array"
              n2461 = property on="data" class="Arr (strict)"() -> ("Value"=w3252:dbl[])  [unwired: 2 in, 2 out]
              n2462 = local read "sweep"() -> (w3257:T3)
              n2463 = Equal?(x=w3257, y=T11."Radio Selection 7" ("sweep")) -> ()  [unwired: 1 out]
              n2464 = case shown="True" FALSE {
                tunnel: [w3260 w3272] -> w3259
                tunnel: [w3261 w3271] -> w3258
                tunnel: w3254 -> [_ w3267]
                tunnel: [_ w3267] -> w3251
                frame True {
                  # "sweeping magnetic field of Hulk"
                  n2465 = stacked-sequence {
                    tunnel: [_ w3263 _] -> w3261
                    tunnel: [_ _ w3265] -> w3260
                    frame #0 {
                      n2466 = local read "Hulk_SMS_addr"() -> (w3262:refnum<visa-resource-name>)
                      n2467 = VISA Clear(VISA resource name=w3262) -> ()  [unwired: 1 in, 2 out]
                    }
                    frame #1 {
                      # "acquires current output value"
                      n2468 = local read "Hulk_SMS_addr"() -> (w3264:refnum<visa-resource-name>)
                      n2469 = call "SMS_GET_OUTPUT.vi"("Hulk_SMS_addr"=w3264) -> ("Numeric"=w3263:dbl)  [unwired: 1 in, 2 out]
                    }
                    frame #2 {
                      # "checks, wheter ramp was finished"
                      n2470 = local read "Hulk_SMS_addr"() -> (w3266:refnum<visa-resource-name>)
                      n2471 = call "SMS_RAMP_STATUS.vi"("Hulk_SMS_addr"=w3266) -> ("selection"=w3265:bool)  [unwired: 1 in, 2 out]
                    }
                  }
                }
                frame False {
                  # "calculate next value"
                  n2472 = property on="sweep to:" class="DigNum (strict)"() -> ("Value"=w3270:dbl)  [unwired: 2 in, 2 out]
                  n2473 = property on="sweep rate, /min" class="DigNum (strict)"() -> ("Value"=w3269:dbl)  [unwired: 2 in, 2 out]
                  n2474 = property on="time/point, sec" class="DigNum (strict)"() -> ("Value"=w3268:dbl)  [unwired: 2 in, 2 out]
                  n2475 = call "CalculateNextValue.vi"("Target a 2"=w3270, "Channel a source value"=w3267, "Ch a sweep rate units/min"=w3269, "time between points, sec"=w3268, "Source a"=Source."Voltage") -> ("Target a"=w3271:dbl, "Boolean"=w3272:bool)
                }
              }
              n2476 = Build Array (concatenate)(w3252, w3251) -> (w3253:dbl[])
              n2477 = property on="data" class="Arr (strict)"("Value"=w3253) -> ()  [unwired: 2 in, 2 out]
            }
            frame #3 {
              n2478 = stacked-sequence "measurement sequence" {
                tunnel: w3274 -> [_ _ _ _ _ _ _ _ _ _ _ _ _ _ _ _ _ _ _ _ _ _ _ _ _ _ w3648 _ _ _ _]
                frame #0 {
                  # "check if in-phase\nsignal on lock-in 1 \nis to be measured"
                  n2479 = property on="data" class="Arr (strict)"() -> ("Value"=w3276:dbl[])  [unwired: 2 in, 2 out]
                  n2480 = local read "SR830 1 ip"() -> (w3275:bool)
                  n2481 = case shown="True" w3275 {
                    tunnel: w3276 -> [w3278 w3287]
                    tunnel: [w3278 w3286] -> w3277
                    frame False {
                      # "we are not measuring in phase signal on lock-in 1 (SR830_1_ip)"
                    }
                    frame True {
                      # "we are  measuring lock-in 1, in phase (SR830_1_ip)"
                      n2482 = local read "SR830 1 addr"() -> (w3280:u8)
                      n2483 = Number To Decimal String(number=w3280) -> (decimal integer string=w3279:string)  [unwired: 1 in]
                      n2484 = GPIB Write(0:w3279, 1:"OUTR?1") -> (6:w3285:errorcluster)  [unwired: 3 in, 1 out]
                      n2485 = GPIB Read(0:w3279, 1:3200, 3:w3285) -> (5:w3283:string)  [unwired: 2 in, 2 out]
                      n2486 = Fract/Exp String To Number(string=w3283) -> (number=w3282:dbl)  [unwired: 3 in, 1 out]
                      n2487 = Build Array (concatenate)(w3287, w3282) -> (w3286:dbl[])
                    }
                  }
                  n2488 = property on="data" class="Arr (strict)"("Value"=w3277) -> ()  [unwired: 2 in, 2 out]
                }
                frame #1 {
                  # "check if out-of-phase\nsignal on lock-in 1 \nis to be measured"
                  n2489 = property on="data" class="Arr (strict)"() -> ("Value"=w3289:dbl[])  [unwired: 2 in, 2 out]
                  n2490 = local read "SR830 1 oop"() -> (w3288:bool)
                  n2491 = case shown="True" w3288 {
                    tunnel: w3289 -> [w3291 w3300]
                    tunnel: [w3291 w3299] -> w3290
                    frame False {
                      # "we are not measuring out of phase signal on lock-in 1 (SR830_1_oop)"
                    }
                    frame True {
                      # "we are  measuring lock-in 1, out of phase (SR830_1_oop)"
                      n2492 = local read "SR830 1 addr"() -> (w3293:u8)
                      n2493 = Number To Decimal String(number=w3293) -> (decimal integer string=w3292:string)  [unwired: 1 in]
                      n2494 = GPIB Write(0:w3292, 1:"OUTR?2") -> (6:w3298:errorcluster)  [unwired: 3 in, 1 out]
                      n2495 = GPIB Read(0:w3292, 1:3200, 3:w3298) -> (5:w3296:string)  [unwired: 2 in, 2 out]
                      n2496 = Fract/Exp String To Number(string=w3296) -> (number=w3295:dbl)  [unwired: 3 in, 1 out]
                      n2497 = Build Array (concatenate)(w3300, w3295) -> (w3299:dbl[])
                    }
                  }
                  n2498 = property on="data" class="Arr (strict)"("Value"=w3290) -> ()  [unwired: 2 in, 2 out]
                }
                frame #2 {
                  # "check if in-phase\nsignal on lock-in 2 \nis to be measured"
                  n2499 = property on="data" class="Arr (strict)"() -> ("Value"=w3302:dbl[])  [unwired: 2 in, 2 out]
                  n2500 = local read "SR830 2 ip"() -> (w3301:bool)
                  n2501 = case shown="True" w3301 {
                    tunnel: w3302 -> [w3304 w3313]
                    tunnel: [w3304 w3312] -> w3303
                    frame False {
                      # "we are not measuring in phase signal on lock-in 2 (SR830_2_ip)"
                    }
                    frame True {
                      # "we are  measuring lock-in 2, in phase (SR830_2_ip)"
                      n2502 = local read "SR830 2 addr"() -> (w3306:u8)
                      n2503 = Number To Decimal String(number=w3306) -> (decimal integer string=w3305:string)  [unwired: 1 in]
                      n2504 = GPIB Write(0:w3305, 1:"OUTP?1") -> (6:w3311:errorcluster)  [unwired: 3 in, 1 out]
                      n2505 = GPIB Read(0:w3305, 1:3200, 3:w3311) -> (5:w3309:string)  [unwired: 2 in, 2 out]
                      n2506 = Fract/Exp String To Number(string=w3309) -> (number=w3308:dbl)  [unwired: 3 in, 1 out]
                      n2507 = Build Array (concatenate)(w3313, w3308) -> (w3312:dbl[])
                    }
                  }
                  n2508 = property on="data" class="Arr (strict)"("Value"=w3303) -> ()  [unwired: 2 in, 2 out]
                }
                frame #3 {
                  # "check if out-of-phase\nsignal on lock-in 2 \nis to be measured"
                  n2509 = property on="data" class="Arr (strict)"() -> ("Value"=w3315:dbl[])  [unwired: 2 in, 2 out]
                  n2510 = local read "SR830 2 oop"() -> (w3314:bool)
                  n2511 = case shown="True" w3314 {
                    tunnel: w3315 -> [w3317 w3326]
                    tunnel: [w3317 w3325] -> w3316
                    frame False {
                      # "we are not measuring out of phase signal on lock-in 2 (SR830_2_oop)"
                    }
                    frame True {
                      # "we are  measuring lock-in 2, out of phase (SR830_2_oop)"
                      n2512 = local read "SR830 2 addr"() -> (w3319:u8)
                      n2513 = Number To Decimal String(number=w3319) -> (decimal integer string=w3318:string)  [unwired: 1 in]
                      n2514 = GPIB Write(0:w3318, 1:"OUTP?2") -> (6:w3324:errorcluster)  [unwired: 3 in, 1 out]
                      n2515 = GPIB Read(0:w3318, 1:3200, 3:w3324) -> (5:w3322:string)  [unwired: 2 in, 2 out]
                      n2516 = Fract/Exp String To Number(string=w3322) -> (number=w3321:dbl)  [unwired: 3 in, 1 out]
                      n2517 = Build Array (concatenate)(w3326, w3321) -> (w3325:dbl[])
                    }
                  }
                  n2518 = property on="data" class="Arr (strict)"("Value"=w3316) -> ()  [unwired: 2 in, 2 out]
                }
                frame #4 {
                  # "check if in-phase\nsignal on lock-in 3 \nis to be measured"
                  n2519 = property on="data" class="Arr (strict)"() -> ("Value"=w3328:dbl[])  [unwired: 2 in, 2 out]
                  n2520 = local read "SR830 3 ip"() -> (w3327:bool)
                  n2521 = case shown="True" w3327 {
                    tunnel: w3328 -> [w3330 w3339]
                    tunnel: [w3330 w3338] -> w3329
                    frame False {
                      # "we are not measuring in phase signal on lock-in 3 (SR830_3_ip)"
                    }
                    frame True {
                      # "we are  measuring lock-in 3, in phase (SR830_3_ip)"
                      n2522 = local read "SR830 3 addr"() -> (w3332:u8)
                      n2523 = Number To Decimal String(number=w3332) -> (decimal integer string=w3331:string)  [unwired: 1 in]
                      n2524 = GPIB Write(0:w3331, 1:"OUTP?1") -> (6:w3337:errorcluster)  [unwired: 3 in, 1 out]
                      n2525 = GPIB Read(0:w3331, 1:3200, 3:w3337) -> (5:w3335:string)  [unwired: 2 in, 2 out]
                      n2526 = Fract/Exp String To Number(string=w3335) -> (number=w3334:dbl)  [unwired: 3 in, 1 out]
                      n2527 = Build Array (concatenate)(w3339, w3334) -> (w3338:dbl[])
                    }
                  }
                  n2528 = property on="data" class="Arr (strict)"("Value"=w3329) -> ()  [unwired: 2 in, 2 out]
                }
                frame #5 {
                  # "check if out-of-phase\nsignal on lock-in 3 \nis to be measured"
                  n2529 = property on="data" class="Arr (strict)"() -> ("Value"=w3341:dbl[])  [unwired: 2 in, 2 out]
                  n2530 = local read "SR830 3 oop"() -> (w3340:bool)
                  n2531 = case shown="True" w3340 {
                    tunnel: w3341 -> [w3343 w3352]
                    tunnel: [w3343 w3351] -> w3342
                    frame False {
                      # "we are not measuring out of phase signal on lock-in 3 (SR830_3_oop)"
                    }
                    frame True {
                      # "we are  measuring lock-in 3, out of phase (SR830_3_oop)"
                      n2532 = local read "SR830 3 addr"() -> (w3345:u8)
                      n2533 = Number To Decimal String(number=w3345) -> (decimal integer string=w3344:string)  [unwired: 1 in]
                      n2534 = GPIB Write(0:w3344, 1:"OUTP?2") -> (6:w3350:errorcluster)  [unwired: 3 in, 1 out]
                      n2535 = GPIB Read(0:w3344, 1:3200, 3:w3350) -> (5:w3348:string)  [unwired: 2 in, 2 out]
                      n2536 = Fract/Exp String To Number(string=w3348) -> (number=w3347:dbl)  [unwired: 3 in, 1 out]
                      n2537 = Build Array (concatenate)(w3352, w3347) -> (w3351:dbl[])
                    }
                  }
                  n2538 = property on="data" class="Arr (strict)"("Value"=w3342) -> ()  [unwired: 2 in, 2 out]
                }
                frame #6 {
                  # "check if in-phase\nsignal on lock-in 4 \nis to be measured"
                  n2539 = property on="data" class="Arr (strict)"() -> ("Value"=w3354:dbl[])  [unwired: 2 in, 2 out]
                  n2540 = local read "SR830 4 ip"() -> (w3353:bool)
                  n2541 = case shown="True" w3353 {
                    tunnel: w3354 -> [w3356 w3365]
                    tunnel: [w3356 w3364] -> w3355
                    frame False {
                      # "we are not measuring in phase signal on lock-in 4 (SR830_4_ip)"
                    }
                    frame True {
                      # "we are  measuring lock-in 4, in phase (SR830_4_ip)"
                      n2542 = local read "SR830 4 addr"() -> (w3358:u8)
                      n2543 = Number To Decimal String(number=w3358) -> (decimal integer string=w3357:string)  [unwired: 1 in]
                      n2544 = GPIB Write(0:w3357, 1:"OUTP?1") -> (6:w3363:errorcluster)  [unwired: 3 in, 1 out]
                      n2545 = GPIB Read(0:w3357, 1:3200, 3:w3363) -> (5:w3361:string)  [unwired: 2 in, 2 out]
                      n2546 = Fract/Exp String To Number(string=w3361) -> (number=w3360:dbl)  [unwired: 3 in, 1 out]
                      n2547 = Build Array (concatenate)(w3365, w3360) -> (w3364:dbl[])
                    }
                  }
                  n2548 = property on="data" class="Arr (strict)"("Value"=w3355) -> ()  [unwired: 2 in, 2 out]
                }
                frame #7 {
                  # "check if out-of-phase\nsignal on lock-in 4 \nis to be measured"
                  n2549 = property on="data" class="Arr (strict)"() -> ("Value"=w3367:dbl[])  [unwired: 2 in, 2 out]
                  n2550 = local read "SR830 4 oop"() -> (w3366:bool)
                  n2551 = case shown="True" w3366 {
                    tunnel: w3367 -> [w3369 w3378]
                    tunnel: [w3369 w3377] -> w3368
                    frame False {
                      # "we are not measuring out of phase signal on lock-in 4 (SR830_4_oop)"
                    }
                    frame True {
                      # "we are  measuring lock-in 4, out of phase (SR830_4_oop)"
                      n2552 = local read "SR830 4 addr"() -> (w3371:u8)
                      n2553 = Number To Decimal String(number=w3371) -> (decimal integer string=w3370:string)  [unwired: 1 in]
                      n2554 = GPIB Write(0:w3370, 1:"OUTP?2") -> (6:w3376:errorcluster)  [unwired: 3 in, 1 out]
                      n2555 = GPIB Read(0:w3370, 1:3200, 3:w3376) -> (5:w3374:string)  [unwired: 2 in, 2 out]
                      n2556 = Fract/Exp String To Number(string=w3374) -> (number=w3373:dbl)  [unwired: 3 in, 1 out]
                      n2557 = Build Array (concatenate)(w3378, w3373) -> (w3377:dbl[])
                    }
                  }
